vi "Log_basic.vi"(8 "errin":errorcluster caption="entrée d'erreur (pas d'erreur)", 9 "date?":bool=TRUE, 10 "chaîne":string, 11 "in":refnum<file>) -> (0 "sortie d'erreur":errorcluster, 3 "refnum en sortie":refnum<file>)   [LabVIEW 2020]
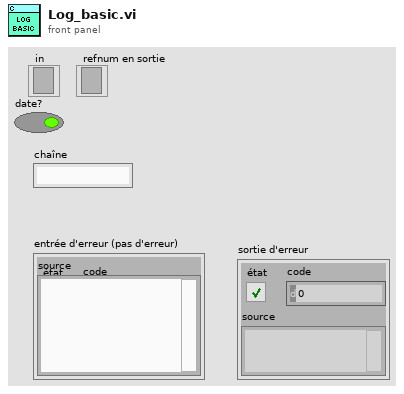
[diagram p1: front panel]
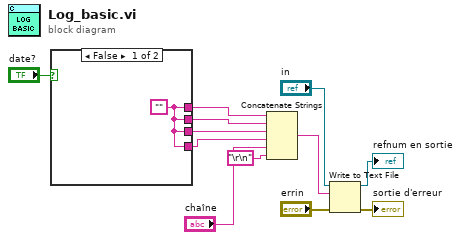
[diagram p0: block diagram]
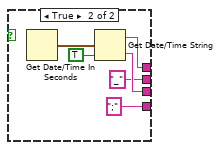
[diagram p2: hidden frame]
diagram:
  n1 = case shown="False" "date?" {
    tunnel: [w13 w19] -> w9
    tunnel: [w13 w18] -> w8
    tunnel: [w13 "_" ("chaîne")] -> w4
    tunnel: [w13 ";" ("chaîne")] -> w1
    frame False {
      w13 = ""
    }
    frame True {
      n2 = Get Date/Time In Seconds() -> (seconds since 1Jan1904=w17:timestamp)
      n3 = Get Date/Time String(seconds (now)=w17, want seconds? (F)=TRUE ("secondes ? (F)")) -> (date string=w18:string, time string=w19:string)  [unwired: 1 in]
    }
  }
  n4 = Concatenate Strings(w8, w4, w9, w1, "chaîne", "\r\n") -> (w5:string)
  n5 = Write to Text File(file (use dialog)="in", text=w5, error in="errin") -> (refnum out=→"refnum en sortie":refnum<file>, error out=→"sortie d'erreur":errorcluster)  [unwired: 1 in, 1 out]
